vi "4 - extract full movement patterns from XY frame and startend frames.vi"() -> ()   [LabVIEW 2013]
uses:
  <vilib>/Utility/file.llb/Read From Spreadsheet File (DBL).vi
panel:
  out "Sub patterns top":string[](array[string])
  out "Sub patterns bottom":string[](array[string])
  in  "file path (dialog if empty) 3":path
  in  "file path (dialog if empty) 2":path
  in  "file path (dialog if empty)":path
  out "top":string[](array[string])
  out "bottom":string[](array[string])
  in  "player transition data":dbl[][](array[numeric])=array14018x2[28036 elements] format="%0.3f"
  in  "startend":dbl[][](array[numeric])=[[400.0, 872.0], [1216.0, 1280.0], [1504.0, 1664.0], [2584.0, 2648.0], [2944.0, 3128.0], [3440.0, 3512.0], [3752.0, 4232.0], [4696.0, 4816.0], [5392.0, 5624.0], [6008.0, 6296.0], [6736.0, 7016.0], [7344.0, 7864.0], [8368.0, 8464.0], [8864.0, 8992.0], [9320.0, 9704.0], [11288.0, 11432.0], [11768.0, 11872.0], [12256.0, 12536.0], [12888.0, 13024.0], [13520.0, 13632.0], [13856.0, 14000.0], [14208.0, 14304.0], [14600.0, 14792.0], [15280.0, 15416.0], [15648.0, 15760.0], [16672.0, 16800.0], [17008.0, 17224.0], [17536.0, 17664.0], [17936.0, 18144.0], [18392.0, 18568.0]] format="%0.3f"
  in  "XY and frame data":dbl[][](array[numeric])=array14019x5[70095 elements] format="%0.3f"
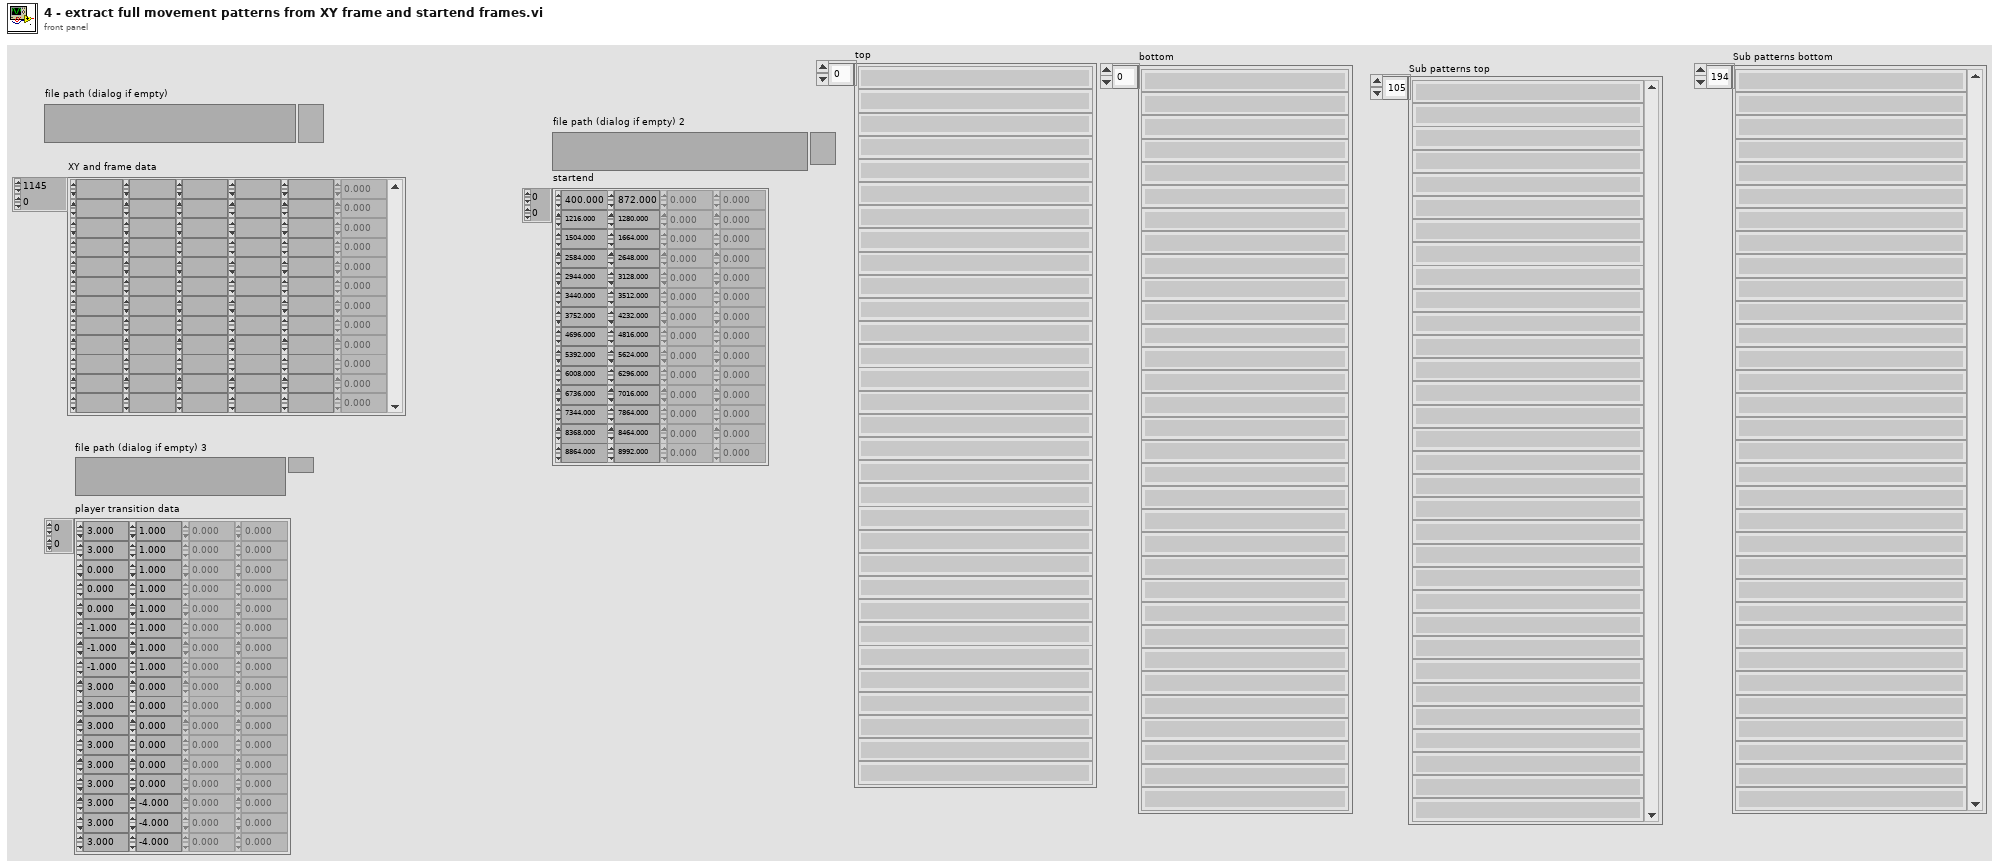
[diagram p1: front panel]
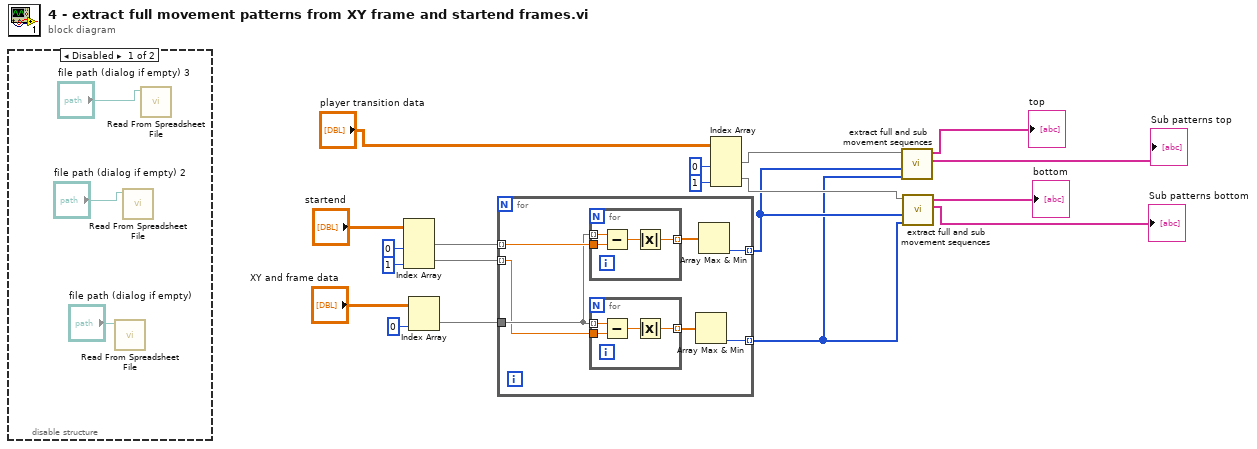
[diagram p0: block diagram]
diagram:
  n1 = disable-structure shown="Disabled" {
    frame Disabled {
      n2 = call-poly <vilib>:"Read From Spreadsheet File.vi"("file path (dialog if empty)"="file path (dialog if empty)") -> ()  [unwired: 6 in, 5 out]
      n3 = call-poly <vilib>:"Read From Spreadsheet File.vi"("file path (dialog if empty)"="file path (dialog if empty) 2") -> ()  [unwired: 6 in, 5 out]
      n4 = call-poly <vilib>:"Read From Spreadsheet File.vi"("file path (dialog if empty)"="file path (dialog if empty) 3") -> ()  [unwired: 6 in, 5 out]
    }
    frame Enabled {
    }
  }
  n5 = Index Array(array="startend", index (col) #1=0 ("disabled index (col)"), index (col) #2=1 ("index (col)")) -> (element #1=w16:dbl[], element #2=w15:dbl[])  [unwired: 2 in]
  n6 = Index Array(array="XY and frame data", index (col)=0 ("disabled index (col)")) -> (element=w12:dbl[])  [unwired: 1 in]
  n7 = for {
    tunnel: w16 -> [w29] mode=indexing
    tunnel: w15 -> [w24] mode=indexing
    tunnel: w12 -> [w25]
    tunnel: [w27] -> w6 mode=indexing
    tunnel: [w26] -> w5 mode=indexing
    n8 = for {
      tunnel: w29 -> [w36]
      tunnel: w25 -> [w37] mode=indexing
      tunnel: [w34] -> w28 mode=indexing
      n9 = Subtract(x=w37, y=w36) -> (x-y=w35:dbl)
      n10 = Absolute Value(x=w35) -> (abs(x)=w34:dbl)
    }
    n11 = for {
      tunnel: w24 -> [w32]
      tunnel: w25 -> [w33] mode=indexing
      tunnel: [w30] -> w23 mode=indexing
      n12 = Subtract(x=w33, y=w32) -> (x-y=w31:dbl)
      n13 = Absolute Value(x=w31) -> (abs(x)=w30:dbl)
    }
    n14 = Array Max & Min(array=w23) -> (min index (indices)=w26:i32)  [unwired: 3 out]
    n15 = Array Max & Min(array=w28) -> (min index (indices)=w27:i32)  [unwired: 3 out]
  }
  n16 = Index Array(array="player transition data", index (col) #1=0 ("disabled index (col)"), index (col) #2=1 ("index (col)")) -> (element #1=w8:dbl[], element #2=w7:dbl[])  [unwired: 2 in]
  n17 = call "extract full and sub movement sequences.vi"("end points in"=w5, "Start points in"=w6, "player movement data"=w8) -> ("Sub patterns"=→"Sub patterns top":string[], "Full movement patterns"=→"top":string[])  [unwired: 7 in]
  n18 = call "extract full and sub movement sequences.vi"("end points in"=w5, "Start points in"=w6, "player movement data"=w7) -> ("Sub patterns"=→"Sub patterns bottom":string[], "Full movement patterns"=→"bottom":string[])  [unwired: 7 in]
